vi "GOOP_CheckIfDependencyViewerCommand.vi"(11 "Command Tag":string) -> (2 "Sub Command":string, 3 "Is It a Dependency Viewer Command":bool)   [LabVIEW 2020]
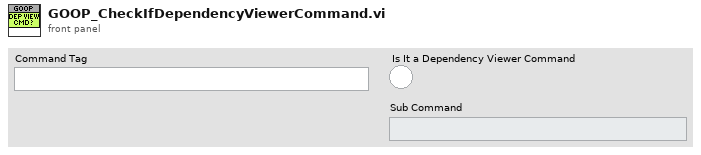
[diagram p1: front panel]
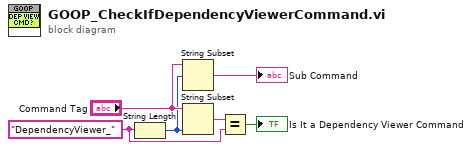
[diagram p0: block diagram]
diagram:
  w5 = "DependencyViewer_" ("Menu Tag")
  n1 = String Length(string=w5) -> (length=w2:i32)
  n2 = String Subset(string="Command Tag", offset (0)=w2) -> (substring=→"Sub Command":string)  [unwired: 1 in]
  n3 = String Subset(string="Command Tag", length (rest)=w2) -> (substring=w4:string)  [unwired: 1 in]
  n4 = Equal?(x=w4, y=w5) -> (x = y?=→"Is It a Dependency Viewer Command":bool)
